vi "Drive_Loop_Initialize.vi"(11 "Name of drive loop (give it a name!)":string) -> (2 "RT FIFO Reference Number":u32, 3 "Drive Loop Cluster":T1)   [LabVIEW 2015]
doc: "Help written by FRC Team 836 - The RoboBees\n\nThis VI creates and intializes the RT FIFOs used in the Chessy Drive drive routines."
uses:
  <userlib>/836-Library/Drive/Drive_Code/Drive_Code_Support/Drive_Code_Bundle.ctl
  <userlib>/836-Library/Drive/Drive_Code/Drive_Code_Support/Sensor_Cluster.ctl
  <userlib>/836-Library/Drive/Drive_Code/Drive_Code_Support/Camera_Cluster.ctl
  <userlib>/836-Library/Drive/Drive_Code/Drive_Code_Support/Drive_Code_Notifier.ctl
  <userlib>/836-Library/Drive/Drive_Code/Drive_Code_Support/Drive_Code_Command.ctl
  <userlib>/836-Library/Drive/Drive_Code/Logging_Data.ctl
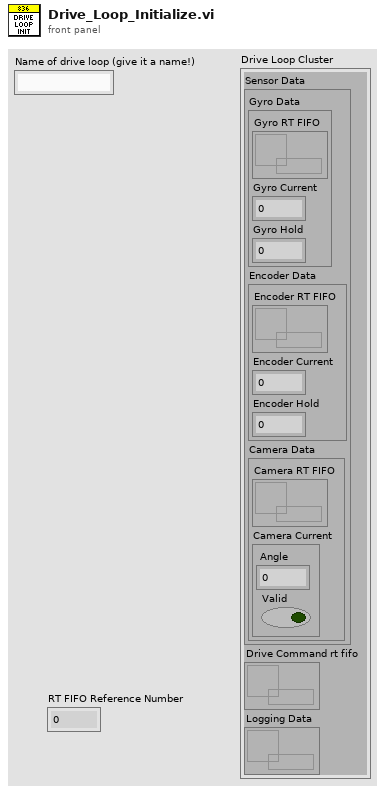
[diagram p1: front panel]
types:
  T1 = typedef "Drive_Code_Bundle.ctl" = cluster{"Sensor Data":T2, "Drive Command rt fifo":refnum<k33>, "Logging Data":refnum<k33>}
  T2 = typedef "Sensor_Cluster.ctl" = cluster{"Gyro Data":cluster{"Gyro RT FIFO":refnum<k33>, "Gyro Current":dbl, "Gyro Hold":dbl}, "Encoder Data":cluster{"Encoder RT FIFO":refnum<k33>, "Encoder Current":dbl, "Encoder Hold":dbl}, "Camera Data":cluster{"Camera RT FIFO":refnum<k33>, "Camera Current":T3}}
  T3 = typedef "Camera_Cluster.ctl" = cluster{" Angle":dbl, "Valid":bool}
  T4 = typedef "Logging_Data.ctl" = cluster{"Command":T5, "Desired Angle":dbl, "Desired Encoder":dbl}
  T5 = typedef "Drive_Code_Command.ctl" = enum16{"Do Nothing", "Manual", "Drive Continuous", "Turn", "Drive Distance", "Hold Position", "Hold Yaw", "Follow Camera", "Turn to Camera"}
  T6 = typedef "Drive_Code_Notifier.ctl" = cluster{"Command":T5, "Parameter A":dbl, "Parameter B":dbl, "Parameter C":dbl, "Absolute?":bool}
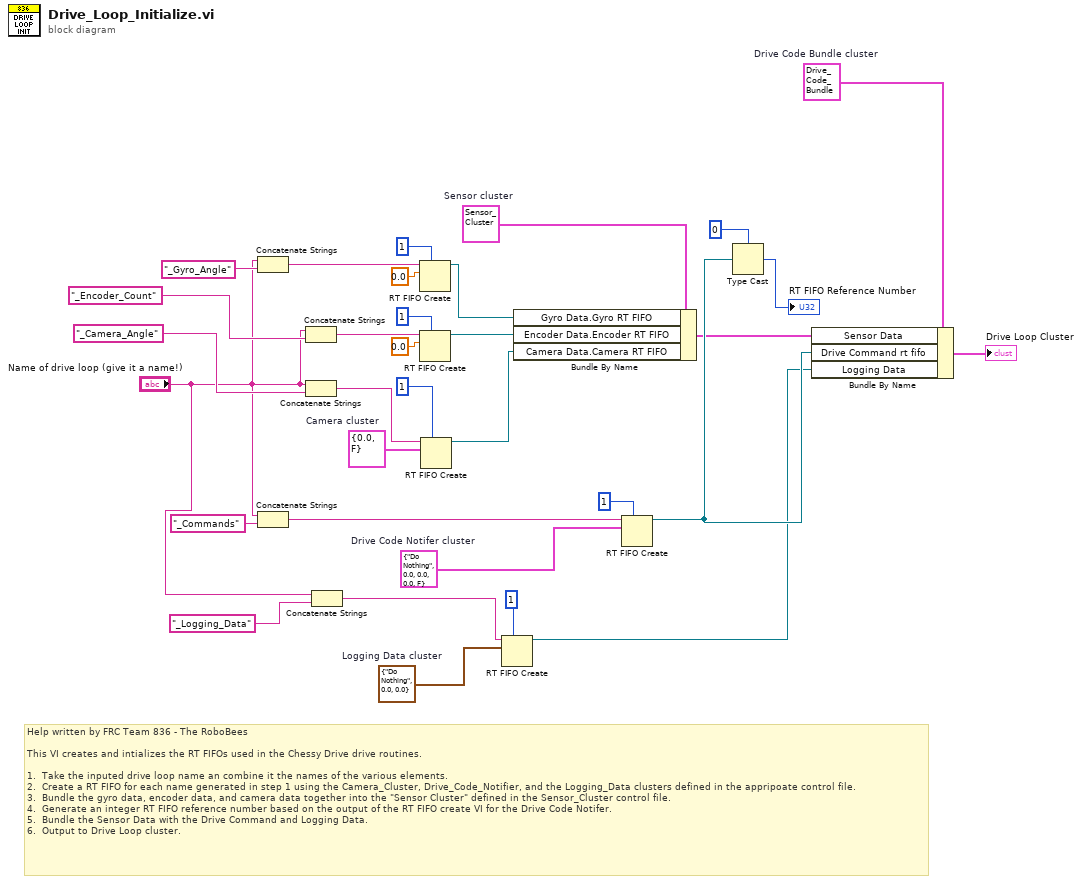
[diagram p0: block diagram]
diagram:
  w6 = T4 {"Command"=enum."Do Nothing", "Desired Angle"=0.0, "Desired Encoder"=0.0}  # Logging Data cluster
  w28 = T1 {"Sensor Data"={"Gyro Data"={"Gyro RT FIFO"=refnum, "Gyro Current"=0.0, "Gyro Hold"=0.0}, "Encoder Data"={"Encoder RT FIFO"=refnum, "Encoder Current"=0.0, "Encoder Hold"=0.0}, "Camera Data"={"Camera RT FIFO"=refnum, "Camera Current"={" Angle"=0.0, "Valid"=FALSE}}}, "Drive Command rt fifo"=refnum, "Logging Data"=refnum}  # Drive Code Bundle cluster
  w26 = T2 {"Gyro Data"={"Gyro RT FIFO"=refnum, "Gyro Current"=0.0, "Gyro Hold"=0.0}, "Encoder Data"={"Encoder RT FIFO"=refnum, "Encoder Current"=0.0, "Encoder Hold"=0.0}, "Camera Data"={"Camera RT FIFO"=refnum, "Camera Current"={" Angle"=0.0, "Valid"=FALSE}}}  # Sensor cluster
  w22 = T3 {" Angle"=0.0, "Valid"=FALSE}  # Camera cluster
  w9 = T6 {"Command"=enum."Do Nothing", "Parameter A"=0.0, "Parameter B"=0.0, "Parameter C"=0.0, "Absolute?"=FALSE}  # Drive Code Notifer cluster
  # "Help written by FRC Team 836 - The RoboBees\n\nThis VI creates and intializes the RT FIFOs used in the Chessy Drive drive routines.\n\n1.  Take the inputed drive loop name an combine it the names of the various elements.\n2.  Create a RT FIFO for each name generated in step 1 using the Camera_Cluster, Drive_Code_Notifier, and the Logging_Data clusters defined in the appripoate control file. \n3.  Bundle the gyro data, encoder data, and camera data together into the \"Sensor Cluster\" defined in the Sensor_Cluster control file. \n4.  Generate an integer RT FIFO reference number based on the output of the RT FIFO create VI for the Drive Code Notifer.\n5.  Bundle the Sensor Data with the Drive Command and Logging Data.\n6.  Output to Drive Loop cluster."
  n1 = Concatenate Strings("Name of drive loop (give it a name!)", "_Gyro_Angle" ("string")) -> (w17:string)
  n2 = Concatenate Strings("Name of drive loop (give it a name!)", "_Commands" ("string")) -> (w8:string)
  n3 = Concatenate Strings("Name of drive loop (give it a name!)", "_Encoder_Count" ("string")) -> (w16:string)
  n4 = Concatenate Strings("Name of drive loop (give it a name!)", "_Camera_Angle" ("string")) -> (w13:string)
  n5 = Concatenate Strings("Name of drive loop (give it a name!)", "_Logging_Data" ("string")) -> (w3:string)
  n6 = RT FIFO Create(0:w17, 1:0.0, 4:u32 1 ("size (10)")) -> (8:w23:refnum<k33>)  [unwired: 5 in, 2 out]
  n7 = RT FIFO Create(0:w16, 1:0.0, 4:u32 1 ("size (10)")) -> (8:w24:refnum<k33>)  [unwired: 5 in, 2 out]
  n8 = RT FIFO Create(0:w13, 1:w22, 4:u32 1 ("size (10)")) -> (8:w25:refnum<k33>)  [unwired: 5 in, 2 out]
  n9 = RT FIFO Create(0:w3, 1:w6, 4:u32 1 ("size (10)")) -> (8:w1:refnum<k33>)  [unwired: 5 in, 2 out]
  n10 = Bundle By Name(cluster=w26, "Gyro Data.Gyro RT FIFO"=w23, "Encoder Data.Encoder RT FIFO"=w24, "Camera Data.Camera RT FIFO"=w25) -> (w27:T2)
  n11 = RT FIFO Create(0:w8, 1:w9, 4:u32 1 ("size (10)")) -> (8:w31:refnum<k33>)  [unwired: 5 in, 2 out]
  n12 = Type Cast(type=u32 0, x=w31) -> (*(type *) &x=→"RT FIFO Reference Number":u32)
  n13 = Bundle By Name(cluster=w28, "Sensor Data"=w27, "Drive Command rt fifo"=w31, "Logging Data"=w1) -> (→"Drive Loop Cluster":T1)
